vi "IMAQDevice.CreateCameraFile.vi"(1 "Ini-File-Path":string, 2 "Camera Name":string, 3 "Attribute Array":cluster{"Command":string, "Value":string}[](array[cluster]), 4 "TimeOut":i32, 5 "error in":errorcluster) -> (15 "File Name":string, 19 "error out":errorcluster)   [LabVIEW 2014, in "IMAQDevice.lvlib"]
uses:
  IMAQDevice.lvlib
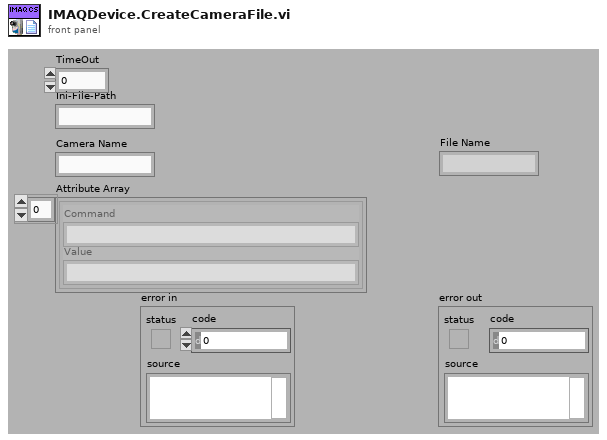
[diagram p1: front panel]
types:
  T1 = enum16{"open", "replace", "create", "open or create", "replace or create", "replace or create with confirmation"}
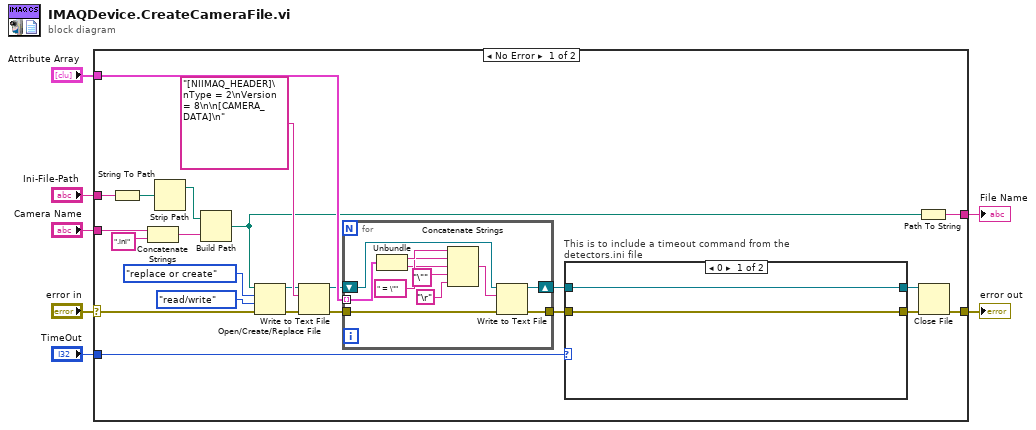
[diagram p0: block diagram]
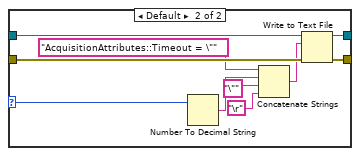
[diagram p2: hidden frame]
diagram:
  n1 = case shown="No Error" "error in" {
    selector: "error in" -> [w21 w54]
    tunnel: "Ini-File-Path" -> [w30 _]
    tunnel: "Camera Name" -> [w24 _]
    tunnel: [w22 w54] -> w5
    tunnel: "Attribute Array" -> [w20 _]
    tunnel: [w13 _] -> w2
    tunnel: "TimeOut" -> [w8 _]
    frame No Error {
      n2 = String To Path(string=w30) -> (path=w29:path)
      n3 = Concatenate Strings(w24, ".ini" ("string")) -> (w25:string)
      n4 = Strip Path(path=w29) -> (stripped path=w26:path)  [unwired: 1 out]
      n5 = Build Path(base path=w26, name or relative path=w25) -> (appended path=w14:path)
      n6 = Open/Create/Replace File(file path (use dialog)=w14, error in=w21, operation (0:open)=T1."replace or create", access (0:read/write)=enum16{"read/write", "read-only", "write-only"}."read/write") -> (refnum out=w18:refnum<file>, error out=w16:errorcluster)  [unwired: 2 in, 1 out]
      n7 = Write to Text File(file (use dialog)=w18, text="[NIIMAQ_HEADER]\nType = 2\nVersion = 8\n\n[CAMERA_DATA]\n", error in=w16) -> (refnum out=w17:refnum<file>, error out=w15:errorcluster)  [unwired: 1 in, 1 out]
      n8 = for {
        tunnel: w15 -> [w53]
        tunnel: [w50] -> w10
        tunnel: w20 -> [w49] mode=indexing
        shift-right: [w51] -> w11
        shift-left: w17 -> [w52]
        n9 = Unbundle(w49) -> ("Command"=w47:string, "Value"=w45:string)
        n10 = Concatenate Strings(w47, " = \"" ("string"), w45, "\"" ("string"), "\r") -> (w48:string)
        n11 = Write to Text File(file (use dialog)=w52, text=w48, error in=w53) -> (refnum out=w51:refnum<file>, error out=w50:errorcluster)  [unwired: 1 in, 1 out]
      }
      n12 = case "This is to include a timeout command from the detectors.ini file" shown="0" w8 {
        selector: w8 -> [_ w34]
        tunnel: [w32 w42] -> w12
        tunnel: w11 -> [w32 w41]
        tunnel: w10 -> [w31 w40]
        tunnel: [w31 w39] -> w9
        frame 0 {
        }
        frame Default {
          n13 = Number To Decimal String(number=w34) -> (decimal integer string=w37:string)  [unwired: 1 in]
          n14 = Concatenate Strings("AcquisitionAttributes::Timeout = \"" ("string"), w37, "\"" ("string"), "\r") -> (w33:string)
          n15 = Write to Text File(file (use dialog)=w41, text=w33, error in=w40) -> (refnum out=w42:refnum<file>, error out=w39:errorcluster)  [unwired: 1 in, 1 out]
        }
      }
      n16 = Path To String(path=w14) -> (string=w13:string)
      n17 = Close File(refnum=w12, error in=w9) -> (error out=w22:errorcluster)  [unwired: 1 out]
    }
    frame Error {
    }
  }
  "error out" <- w5
  "File Name" <- w2
